vi "array_size.vi"(0 "Array":dbl[][](array[numeric]), 1 "Dimension":i32) -> (5 "Dimension size":i32)   [LabVIEW 2011, in "Fiberscope_library.lvlib"]
doc: "Returns the size of dimension [Dimension] of the input array [Array]. 0: rows, 1: columns, ..."
uses:
  Fiberscope_library.lvlib
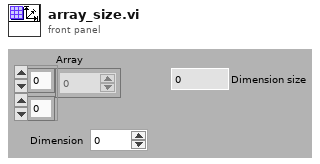
[diagram p1: front panel]
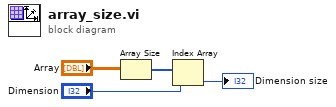
[diagram p0: block diagram]
diagram:
  n1 = Array Size(array="Array") -> (size(s)=w2:i32[])
  n2 = Index Array(array=w2, index="Dimension") -> (element=→"Dimension size":i32)
